vi "RANGE Select Meter.vi"(6 "Rate Threshold (V)":dbl, 8 "Error In":errorcluster, 9 "Meter Number":T7, 10 "All Meter Data":T1={"Meter 1"={"Meter Size"=0.0, "DAQ Output (Voltage)"=0.0, "Reference (Voltage)"=0.0, "Meter Present"=FALSE, "Meter Visa"="", "Gas Type"="", "SLPM Error @ Zero"=0.0, "Gas Mix Number"="", "Set STP Register"=FALSE}, "Meter 2"={"Meter Size"=0.0, "DAQ Output (Voltage)"=0.0, "Reference (Voltage)"=0.0, "Meter Present"=FALSE, "Meter Visa"="", "Gas Type"="", "SLPM Error @ Zero"=0.0, "Gas Mix Number"="", "Set STP Register"=FALSE}, "Meter 3"={"Meter Size"=0.0, "DAQ Output (Voltage)"=0.0, "Reference (Voltage)"=0.0, "Meter Present"=FALSE, "Meter Visa"="", "Gas Type"="", "SLPM Error @ Zero"=0.0, "Gas Mix Number"="", "Set STP Register"=FALSE}, "Meter 4"={"Meter Size"=0.0, "DAQ Output (Voltage)"=0.0, "Reference (Voltage)"=0.0, "Meter Present"=FALSE, "Meter Visa"="", "Gas Type"="", "SLPM Error @ Zero"=0.0, "Gas Mix Number"="", "Set STP Register"=FALSE}, "Meter 5"={"Meter Size"=0.0, "DAQ Output (Voltage)"=0.0, "Reference (Voltage)"=0.0, "Meter Present"=FALSE, "Meter Visa"="", "Gas Type"="", "SLPM Error @ Zero"=0.0, "Gas Mix Number"="", "Set STP Register"=FALSE}, "Meter 6"={"Meter Size"=0.0, "DAQ Output (Voltage)"=0.0, "Reference (Voltage)"=0.0, "Meter Present"=FALSE, "Meter Visa"="", "Gas Type"="", "SLPM Error @ Zero"=0.0, "Gas Mix Number"="", "Set STP Register"=FALSE}, "Meter Bank 1"={"Flow Rate (BTU/HR)"=0.0, "ANSI Placeholder Array"=[], "15 Sec Avg Array"=[], "30 Sec Avg Array "=[], "ANSI Average (BTU/HR)"=0.0, "Panel Data"={"Meter Type (Gas)"="", "Meter ID"=enum."Disabled", "Heating Value (BTU/ft³)"=0.0, "Ft³ / Hr (SCFH)"=0.0, "15 Second Average (BTU/HR)"=0.0, "30 Second Average (BTU/HR)"=0.0, "SLPM (Mass Flow)"=0.0, "LPM (Vol. Flow)"=0.0, "Gas Temperature (°F)"=0.0, "Gas Pressure (PSIA)"=0.0, "Tot.Flow (Liters)"=0.0}, "Start ANSI"=FALSE, "ANSI Start Time"=0.0, "Restart ANSI"=FALSE}, "Meter Bank 2"={"Flow Rate (BTU/HR)"=0.0, "ANSI Placeholder Array"=[], "15 Sec Avg Array"=[], "30 Sec Avg Array "=[], "ANSI Average (BTU/HR)"=0.0, "Panel Data"={"Meter Type (Gas)"="", "Meter ID"=enum."Disabled", "Heating Value (BTU/ft³)"=0.0, "Ft³ / Hr (SCFH)"=0.0, "15 Second Average (BTU/HR)"=0.0, "30 Second Average (BTU/HR)"=0.0, "SLPM (Mass Flow)"=0.0, "LPM (Vol. Flow)"=0.0, "Gas Temperature (°F)"=0.0, "Gas Pressure (PSIA)"=0.0, "Tot.Flow (Liters)"=0.0}, "Start ANSI"=FALSE, "ANSI Start Time"=0.0, "Restart ANSI"=FALSE}, "Meter Bank 3"={"Flow Rate (BTU/HR)"=0.0, "ANSI Placeholder Array"=[], "15 Sec Avg Array"=[], "30 Sec Avg Array "=[], "ANSI Average (BTU/HR)"=0.0, "Panel Data"={"Meter Type (Gas)"="", "Meter ID"=enum."Disabled", "Heating Value (BTU/ft³)"=0.0, "Ft³ / Hr (SCFH)"=0.0, "15 Second Average (BTU/HR)"=0.0, "30 Second Average (BTU/HR)"=0.0, "SLPM (Mass Flow)"=0.0, "LPM (Vol. Flow)"=0.0, "Gas Temperature (°F)"=0.0, "Gas Pressure (PSIA)"=0.0, "Tot.Flow (Liters)"=0.0}, "Start ANSI"=FALSE, "ANSI Start Time"=0.0, "Restart ANSI"=FALSE}, "Threshold Voltage (NI DAQ)"=0.2, "Use RS232 Data Collection"=FALSE}) -> (0 "Error Out":errorcluster, 2 "All Meter Data Out":T1={"Meter 1"={"Meter Size"=0.0, "DAQ Output (Voltage)"=0.0, "Reference (Voltage)"=0.0, "Meter Present"=FALSE, "Meter Visa"="", "Gas Type"="", "SLPM Error @ Zero"=0.0, "Gas Mix Number"="", "Set STP Register"=FALSE}, "Meter 2"={"Meter Size"=0.0, "DAQ Output (Voltage)"=0.0, "Reference (Voltage)"=0.0, "Meter Present"=FALSE, "Meter Visa"="", "Gas Type"="", "SLPM Error @ Zero"=0.0, "Gas Mix Number"="", "Set STP Register"=FALSE}, "Meter 3"={"Meter Size"=0.0, "DAQ Output (Voltage)"=0.0, "Reference (Voltage)"=0.0, "Meter Present"=FALSE, "Meter Visa"="", "Gas Type"="", "SLPM Error @ Zero"=0.0, "Gas Mix Number"="", "Set STP Register"=FALSE}, "Meter 4"={"Meter Size"=0.0, "DAQ Output (Voltage)"=0.0, "Reference (Voltage)"=0.0, "Meter Present"=FALSE, "Meter Visa"="", "Gas Type"="", "SLPM Error @ Zero"=0.0, "Gas Mix Number"="", "Set STP Register"=FALSE}, "Meter 5"={"Meter Size"=0.0, "DAQ Output (Voltage)"=0.0, "Reference (Voltage)"=0.0, "Meter Present"=FALSE, "Meter Visa"="", "Gas Type"="", "SLPM Error @ Zero"=0.0, "Gas Mix Number"="", "Set STP Register"=FALSE}, "Meter 6"={"Meter Size"=0.0, "DAQ Output (Voltage)"=0.0, "Reference (Voltage)"=0.0, "Meter Present"=FALSE, "Meter Visa"="", "Gas Type"="", "SLPM Error @ Zero"=0.0, "Gas Mix Number"="", "Set STP Register"=FALSE}, "Meter Bank 1"={"Flow Rate (BTU/HR)"=0.0, "ANSI Placeholder Array"=[], "15 Sec Avg Array"=[], "30 Sec Avg Array "=[], "ANSI Average (BTU/HR)"=0.0, "Panel Data"={"Meter Type (Gas)"="", "Meter ID"=enum."Disabled", "Heating Value (BTU/ft³)"=0.0, "Ft³ / Hr (SCFH)"=0.0, "15 Second Average (BTU/HR)"=0.0, "30 Second Average (BTU/HR)"=0.0, "SLPM (Mass Flow)"=0.0, "LPM (Vol. Flow)"=0.0, "Gas Temperature (°F)"=0.0, "Gas Pressure (PSIA)"=0.0, "Tot.Flow (Liters)"=0.0}, "Start ANSI"=FALSE, "ANSI Start Time"=0.0, "Restart ANSI"=FALSE}, "Meter Bank 2"={"Flow Rate (BTU/HR)"=0.0, "ANSI Placeholder Array"=[], "15 Sec Avg Array"=[], "30 Sec Avg Array "=[], "ANSI Average (BTU/HR)"=0.0, "Panel Data"={"Meter Type (Gas)"="", "Meter ID"=enum."Disabled", "Heating Value (BTU/ft³)"=0.0, "Ft³ / Hr (SCFH)"=0.0, "15 Second Average (BTU/HR)"=0.0, "30 Second Average (BTU/HR)"=0.0, "SLPM (Mass Flow)"=0.0, "LPM (Vol. Flow)"=0.0, "Gas Temperature (°F)"=0.0, "Gas Pressure (PSIA)"=0.0, "Tot.Flow (Liters)"=0.0}, "Start ANSI"=FALSE, "ANSI Start Time"=0.0, "Restart ANSI"=FALSE}, "Meter Bank 3"={"Flow Rate (BTU/HR)"=0.0, "ANSI Placeholder Array"=[], "15 Sec Avg Array"=[], "30 Sec Avg Array "=[], "ANSI Average (BTU/HR)"=0.0, "Panel Data"={"Meter Type (Gas)"="", "Meter ID"=enum."Disabled", "Heating Value (BTU/ft³)"=0.0, "Ft³ / Hr (SCFH)"=0.0, "15 Second Average (BTU/HR)"=0.0, "30 Second Average (BTU/HR)"=0.0, "SLPM (Mass Flow)"=0.0, "LPM (Vol. Flow)"=0.0, "Gas Temperature (°F)"=0.0, "Gas Pressure (PSIA)"=0.0, "Tot.Flow (Liters)"=0.0}, "Start ANSI"=FALSE, "ANSI Start Time"=0.0, "Restart ANSI"=FALSE}, "Threshold Voltage (NI DAQ)"=0.2, "Use RS232 Data Collection"=FALSE})   [LabVIEW 2016]
uses:
  Type Definitions/Range Meter Bank.ctl
  Type Definitions/RANGE DAQ Data Four Meters.ctl
  Type Definitions/RANGE DAQ Data.ctl
  Drivers/Omega FMA-1600A Series Gas Flow Meter/Type Definitions/FMA1600A Gas Type.ctl
  Type Definitions/RANGE GAS Data.ctl
  Type Definitions/RANGE Panel Data.ctl
  Type Definitions/RANGE Meter Selector 1-2.ctl
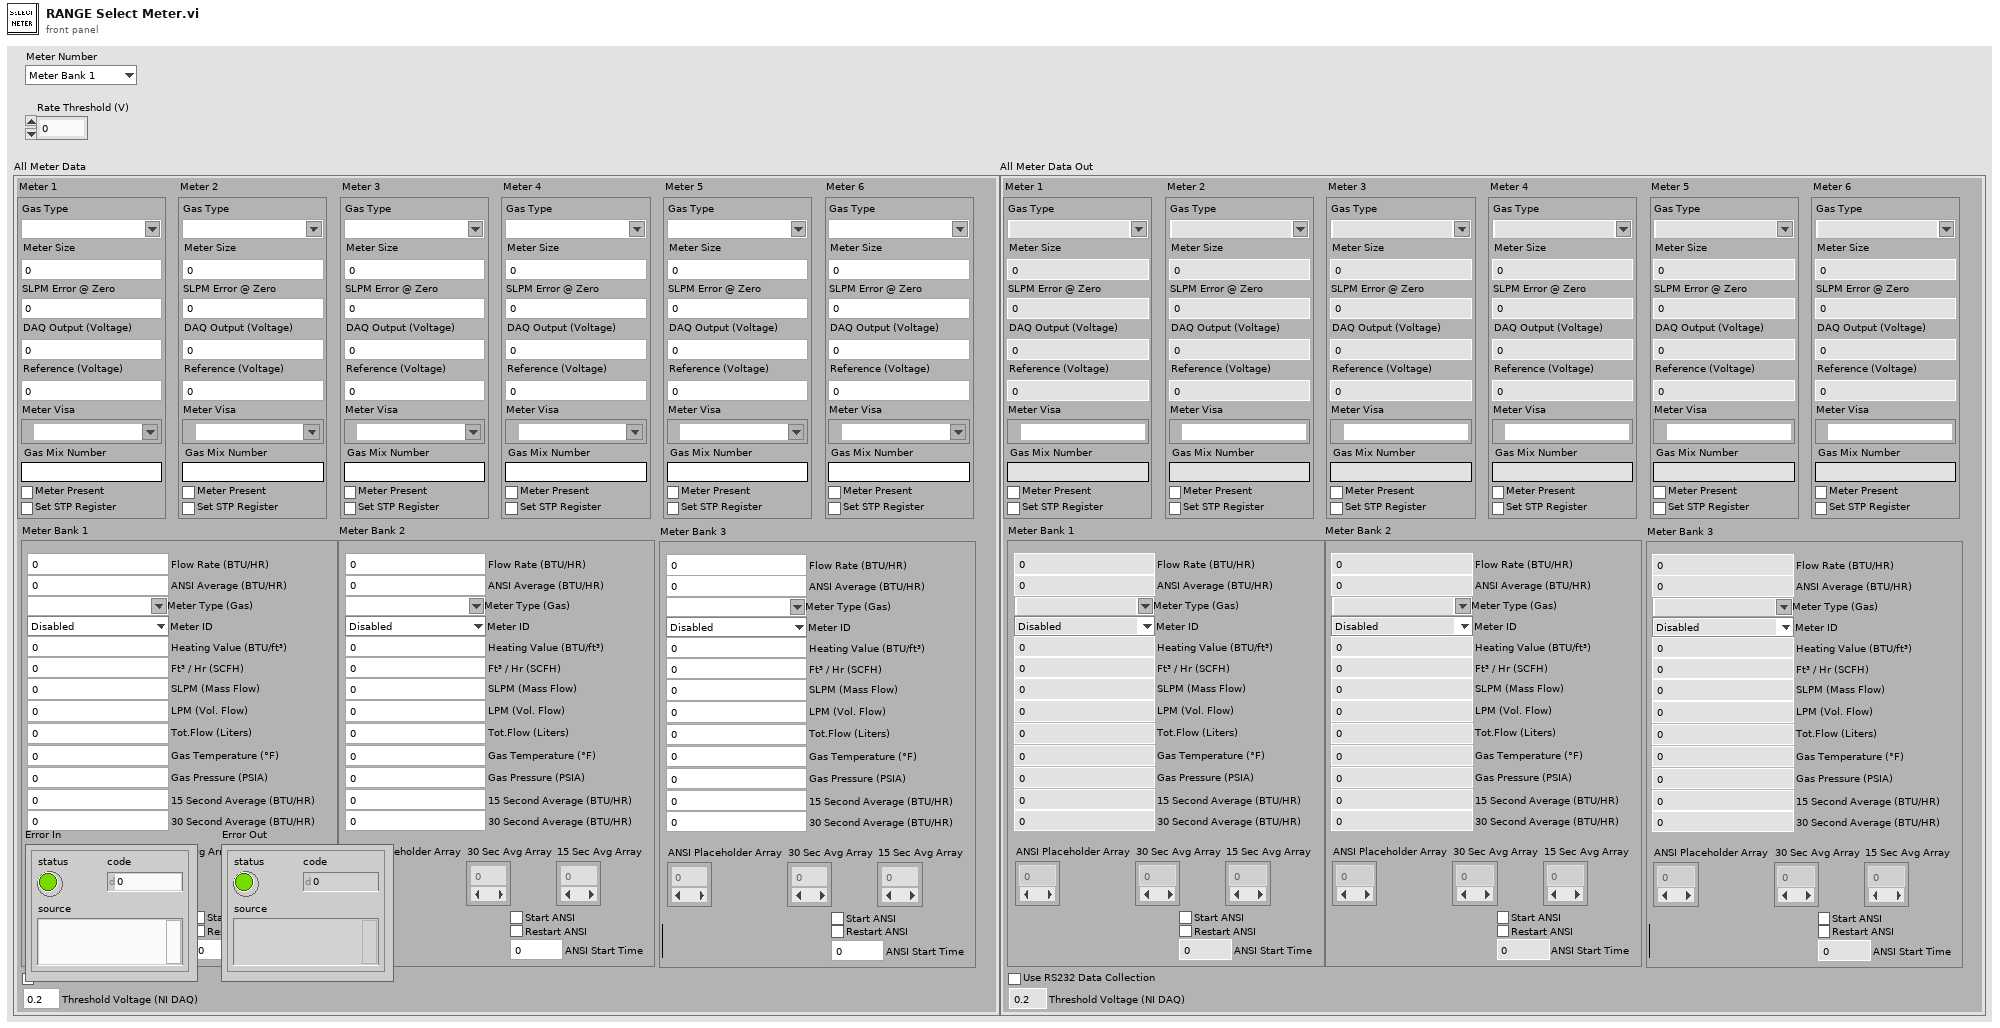
[diagram p1: front panel]
types:
  T1 = typedef "RANGE DAQ Data Four Meters.ctl" = cluster{"Meter 1":T2, "Meter 2":T2, "Meter 3":T2, "Meter 4":T2, "Meter 5":T2, "Meter 6":T2, "Meter Bank 1":T4, "Meter Bank 2":T4, "Meter Bank 3":T4, "Threshold Voltage (NI DAQ)":dbl, "Use RS232 Data Collection":bool}
  T2 = typedef "RANGE DAQ Data.ctl" = cluster{"Meter Size":dbl, "DAQ Output (Voltage)":dbl, "Reference (Voltage)":dbl, "Meter Present":bool, "Meter Visa":refnum<visa-resource-name>, "Gas Type":T3, "SLPM Error @ Zero":dbl, "Gas Mix Number":string, "Set STP Register":bool}
  T3 = typedef "FMA1600A Gas Type.ctl" = string
  T4 = typedef "RANGE GAS Data.ctl" = cluster{"Flow Rate (BTU/HR)":dbl, "ANSI Placeholder Array":dbl[], "15 Sec Avg Array":dbl[], "30 Sec Avg Array ":dbl[], "ANSI Average (BTU/HR)":dbl, "Panel Data":T5, "Start ANSI":bool, "ANSI Start Time":dbl, "Restart ANSI":bool}
  T5 = typedef "RANGE Panel Data.ctl" = cluster{"Meter Type (Gas)":T3, "Meter ID":T6, "Heating Value (BTU/ft³)":dbl, "Ft³ / Hr (SCFH)":dbl, "15 Second Average (BTU/HR)":dbl, "30 Second Average (BTU/HR)":dbl, "SLPM (Mass Flow)":dbl, "LPM (Vol. Flow)":dbl, "Gas Temperature (°F)":dbl, "Gas Pressure (PSIA)":dbl, "Tot.Flow (Liters)":dbl}
  T6 = typedef "RANGE Meter Selector 1-2.ctl" = enum16{"Disabled", "Small", "Large"}
  T7 = typedef "Range Meter Bank.ctl" = enum16{"Meter Bank 1", "Meter Bank 2", "Meter Bank 3"}
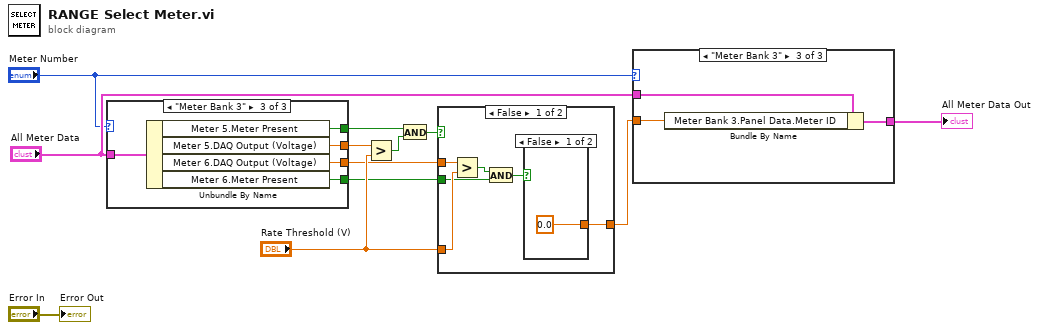
[diagram p0: block diagram]
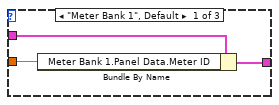
[diagram p2: hidden frame]
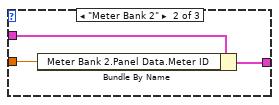
[diagram p3: hidden frame]
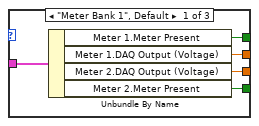
[diagram p4: hidden frame]
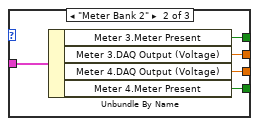
[diagram p5: hidden frame]
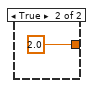
[diagram p6: hidden frame]
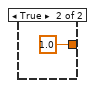
[diagram p7: hidden frame]
diagram:
  n1 = case shown="\"Meter Bank 3\"" "Meter Number" {
    tunnel: "All Meter Data" -> [w17 w22 w27]
    tunnel: [w16 w21 w26] -> w10
    tunnel: [w15 w20 w25] -> w11
    tunnel: [w13 w18 w24] -> w6
    tunnel: [w14 w19 w23] -> w7
    frame "Meter Bank 1", Default {
      n2 = Unbundle By Name(w17) -> ("Meter 1.Meter Present"=w14:bool, "Meter 1.DAQ Output (Voltage)"=w16:dbl, "Meter 2.DAQ Output (Voltage)"=w15:dbl, "Meter 2.Meter Present"=w13:bool)
    }
    frame "Meter Bank 2" {
      n3 = Unbundle By Name(w22) -> ("Meter 3.Meter Present"=w19:bool, "Meter 3.DAQ Output (Voltage)"=w21:dbl, "Meter 4.DAQ Output (Voltage)"=w20:dbl, "Meter 4.Meter Present"=w18:bool)
    }
    frame "Meter Bank 3" {
      n4 = Unbundle By Name(w27) -> ("Meter 5.Meter Present"=w23:bool, "Meter 5.DAQ Output (Voltage)"=w26:dbl, "Meter 6.DAQ Output (Voltage)"=w25:dbl, "Meter 6.Meter Present"=w24:bool)
    }
  }
  n5 = Greater?(x=w10, y="Rate Threshold (V)") -> (0:w8:bool)
  n6 = And(x=w7, y=w8) -> (x .and. y?=w9:bool)
  n7 = case shown="False" w9 {
    tunnel: w11 -> [w31 _]
    tunnel: "Rate Threshold (V)" -> [w30 _]
    tunnel: [w29 1.0] -> w1
    tunnel: w6 -> [w28 _]
    frame False {
      n8 = Greater?(x=w31, y=w30) -> (0:w33:bool)
      n9 = And(x=w33, y=w28) -> (x .and. y?=w32:bool)
      n10 = case shown="False" w32 {
        tunnel: [0.0 2.0] -> w29
        frame False {
        }
        frame True {
        }
      }
    }
    frame True {
    }
  }
  n11 = case shown="\"Meter Bank 3\"" "Meter Number" {
    tunnel: "All Meter Data" -> [w39 w41 w45]
    tunnel: [w38 w40 w44] -> w2
    tunnel: w1 -> [w37 w42 w43]
    frame "Meter Bank 1", Default {
      n12 = Bundle By Name(cluster=w39, "Meter Bank 1.Panel Data.Meter ID"=w37) -> (w38:T1)
    }
    frame "Meter Bank 2" {
      n13 = Bundle By Name(cluster=w41, "Meter Bank 2.Panel Data.Meter ID"=w42) -> (w40:T1)
    }
    frame "Meter Bank 3" {
      n14 = Bundle By Name(cluster=w45, "Meter Bank 3.Panel Data.Meter ID"=w43) -> (w44:T1)
    }
  }
  "All Meter Data Out" <- w2
  "Error Out" <- "Error In"
